vi "VD-getDeviceInfo.vi"(8 "error in (no error)":errorcluster, 11 "VD-LV-LiteVNA in":refnum<class "VD-LV-LiteVNA.lvclass">) -> (0 "error out":errorcluster, 2 "device info":T1, 3 "VD-LV-LiteVNA out":refnum<class "VD-LV-LiteVNA.lvclass">)   [LabVIEW 2020, in "VD-LV-LiteVNA.lvclass"]
uses:
  VD-LV-LiteVNA.lvclass
  VD-device_info.ctl
  VD-action.ctl
  VD-LV-LiteVNA.lvclass/VD-LV-LiteVNA.ctl
  hardware-protocol/serial/HP-S-Serial.lvclass
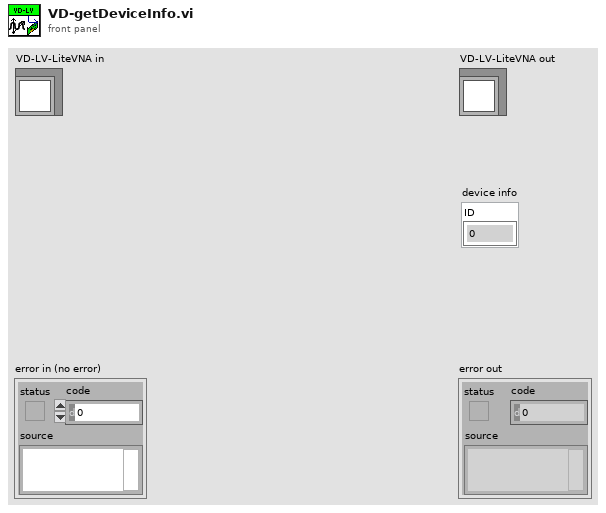
[diagram p1: front panel]
types:
  T1 = typedef "VD-LV-LiteVNA.lvclass/VD-device_info.ctl" = cluster{"ID":u8}
  T2 = typedef "VD-LV-LiteVNA.lvclass/VD-action.ctl" = enum16{"checkCom", "SweepStartHz", "SweepStopHz", "SweepPoints", "valuesPerFrequency", "RawSamplesMode", "ValuesFIFO", "deviceVariant", "protocolVersion", "hardwareRevision", "firmwareMajor", "firmwareMinor"}
  T3 = typedef "HP-S-Serial.lvclass/HP-S-data.ctl" = u8[]
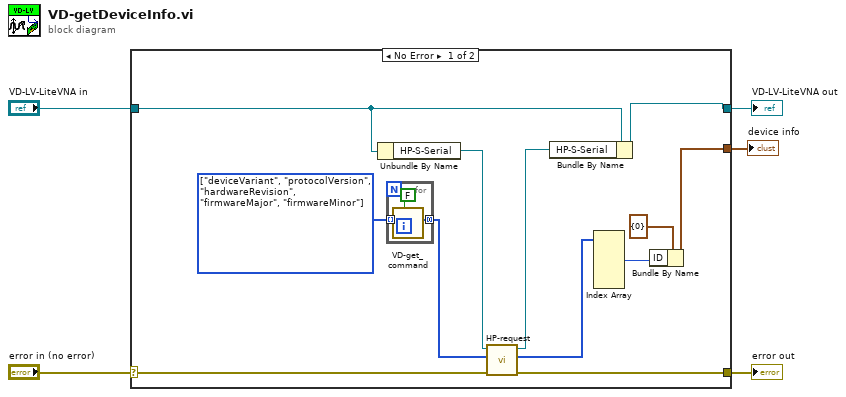
[diagram p0: block diagram]
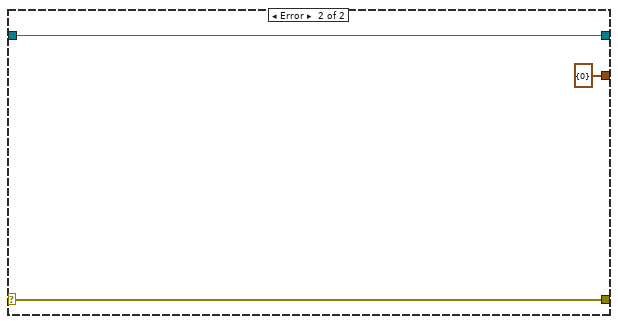
[diagram p2: hidden frame]
diagram:
  n1 = case shown="No Error" "error in (no error)" {
    selector: "error in (no error)" -> [w11 w23]
    tunnel: [w10 w23] -> w4
    tunnel: [w12 w22] -> w2
    tunnel: "VD-LV-LiteVNA in" -> [w13 w22]
    tunnel: [w7 T1 {"ID"=0} ("device info")] -> w1
    frame No Error {
      w16 = T2[] [enum."deviceVariant", enum."protocolVersion", enum."hardwareRevision", enum."firmwareMajor", enum."firmwareMinor"] items=["checkCom", "SweepStartHz", "SweepStopHz", "SweepPoints", "valuesPerFrequency", "RawSamplesMode", "ValuesFIFO", "deviceVariant", "protocolVersion", "hardwareRevision", "firmwareMajor", "firmwareMinor"] ("Array")
      n2 = Unbundle By Name(w13) -> ("HP-S-Serial"=w15:refnum<class "HP-S-Serial.lvclass">)
      n3 = for {
        tunnel: [w20] -> w17 mode=concatenating
        tunnel: w16 -> [w19] mode=indexing
        n4 = call "VD-get_command.vi"("Write?"=FALSE, "action"=w19) -> ("Command"=w20:T3)  [unwired: 9 in]
      }
      n5 = call-dynamic "HP-request.vi"("error in (no error)"=w11, "write buffer"=w17, "HP-S-Serial in"=w15) -> ("error out"=w10:errorcluster, "read buffer"=w9:T3, "HP-S-Serial out"=w14:refnum<class "HP-S-Serial.lvclass">)  [unwired: 6 in]
      n6 = Bundle By Name(cluster=w13, "HP-S-Serial"=w14) -> (w12:refnum<class "VD-LV-LiteVNA.lvclass">)
      n7 = Index Array(array=w9) -> (element #2=w6:u8)  [unwired: 5 in, 4 out]
      n8 = Bundle By Name(cluster=T1 {"ID"=0} ("device info"), "ID"=w6) -> (w7:T1)
    }
    frame Error {
    }
  }
  "error out" <- w4
  "VD-LV-LiteVNA out" <- w2
  "device info" <- w1
